vi "HexStringToASCII.vi"(10 "HexIStringnput":string="523135313230303737342C523135313230303734362C52313531323030373135") -> (2 "AsciiOutput":string)   [LabVIEW 2012]
panel:
  out "substring":string
  out "x/y":dbl
  out "number":u32
  out "*(type *) &x":string
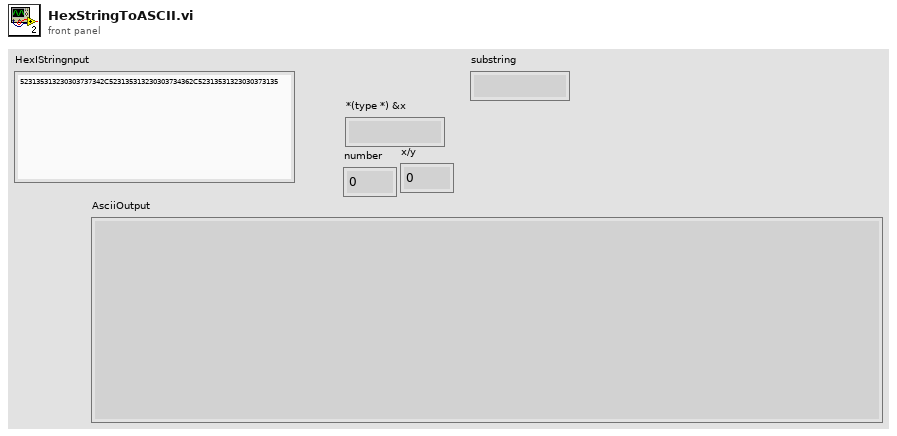
[diagram p1: front panel]
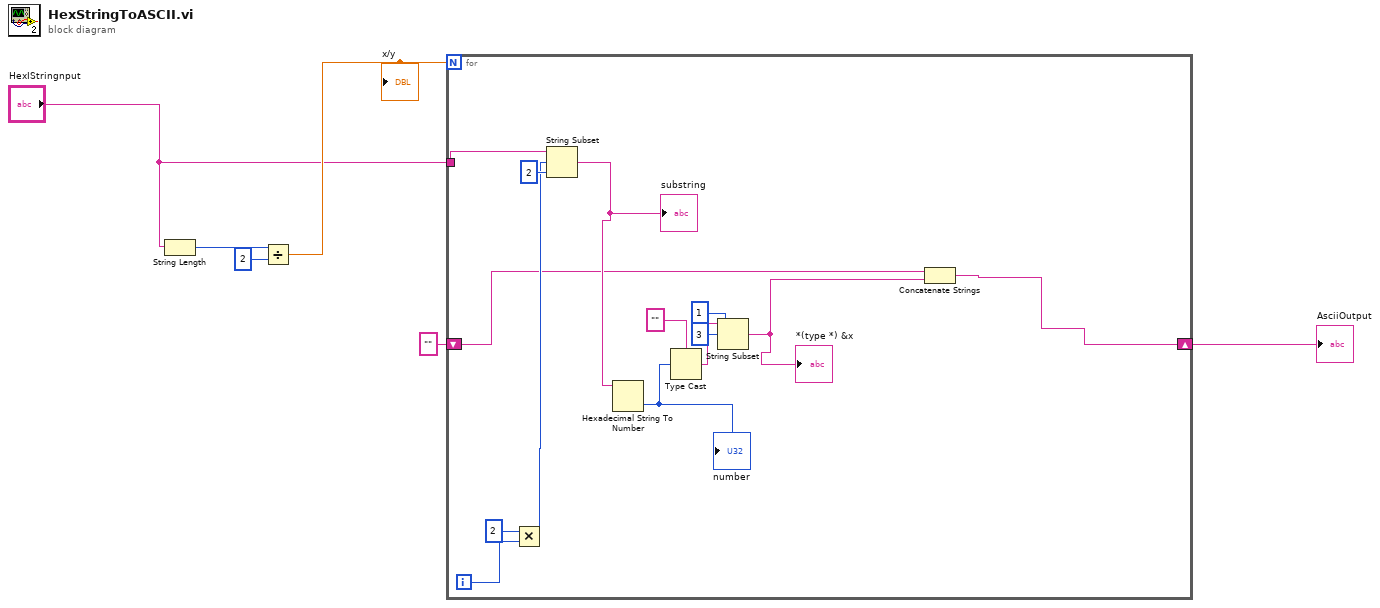
[diagram p0: block diagram]
diagram:
  n1 = String Length(string="HexIStringnput") -> (length=w6:i32)
  n2 = Divide(x=w6, y=2) -> (x/y=w4:dbl)
  "x/y" <- w4
  n3 = for {
    N: w4 -> [_]
    tunnel: "HexIStringnput" -> [w19]
    shift-right: [w7] -> w2
    shift-left: "" -> [w8]
    i -> [w17]
    n4 = Multiply(x=2, y=w17) -> (x*y=w15:i32)
    n5 = String Subset(string=w19, offset (0)=w15, length (rest)=2 ("length (rest)")) -> (substring=w14:string)
    "substring" <- w14
    n6 = Hexadecimal String To Number(string=w14) -> (number=w20:u32)  [unwired: 2 in, 1 out]
    "number" <- w20
    n7 = Type Cast(type="", x=w20) -> (*(type *) &x=w12:string)
    n8 = String Subset(string=w12, offset (0)=3, length (rest)=1 ("length (rest)")) -> (substring=w9:string)
    "*(type *) &x" <- w9
    n9 = Concatenate Strings(w8, w9) -> (w7:string)
  }
  "AsciiOutput" <- w2
